vi "Deep Search Priv.vi"(0 "Tree Dictionary In":variant, 5 "Name":string, 11 "error in":errorcluster) -> (4 "Tree Dictionary Out":variant, 6 "IDs":string[](array[string]), 15 "error out":errorcluster)   [LabVIEW 2016, in "Tree Manager.lvclass"]
uses:
  Tree Manager.lvclass
  Typedefs/Tree.ctl
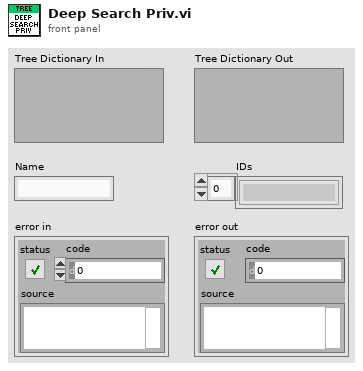
[diagram p1: front panel]
types:
  T1 = typedef "Tree Manager.lvclass/Tree.ctl" = cluster{"Unique ID":string, "Parent ID":string, "Child IDs":string[], "Data":variant, "Name":string}
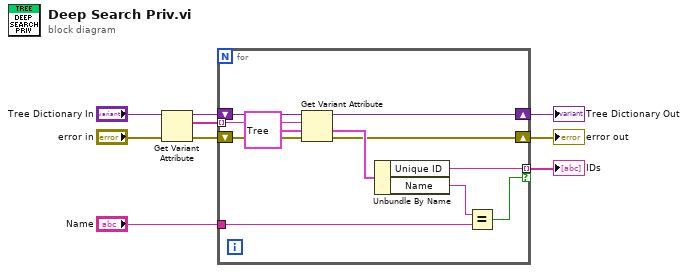
[diagram p0: block diagram]
diagram:
  n1 = Get Variant Attribute(Variant="Tree Dictionary In", error in="error in") -> (duplicate Variant=w1:variant, names=w7:string[], error out=w8:errorcluster)  [unwired: 2 in, 1 out]
  n2 = for {
    tunnel: "Name" -> [w18]
    shift-right: [w14] -> w3
    shift-left: w1 -> [w20]
    tunnel: [w13] -> w6 mode=indexing if=w12
    shift-right: [w15] -> w4
    shift-left: w8 -> [w16]
    tunnel: w7 -> [w11] mode=indexing
    n3 = Get Variant Attribute(Variant=w20, name=w11, default value (empty Variant)=T1 {"Unique ID"="", "Parent ID"="", "Child IDs"=[], "Data"=variant, "Name"=""} ("Cluster of class private data"), error in=w16) -> (duplicate Variant=w14:variant, value=w19:T1, error out=w15:errorcluster)  [unwired: 1 out]
    n4 = Unbundle By Name(w19) -> ("Unique ID"=w13:string, "Name"=w17:string)
    n5 = Equal?(x=w17, y=w18) -> (x = y?=w12:bool)
  }
  "IDs" <- w6
  "error out" <- w4
  "Tree Dictionary Out" <- w3
